vi "Write Start URL.vi"(8 "error in (no error)":errorcluster, 10 "Start URL":string, 11 "WebView2 Control in":refnum<class "WebView2 Control.lvclass">) -> (0 "error out":errorcluster, 3 "WebView2 Control out":refnum<class "WebView2 Control.lvclass">)   [LabVIEW 2020, in "WebView2.lvlib" / "WebView2 Control.lvclass"]
uses:
  WebView2 Control.lvclass
  WebView2 Control.lvclass/WebView2 Control.ctl
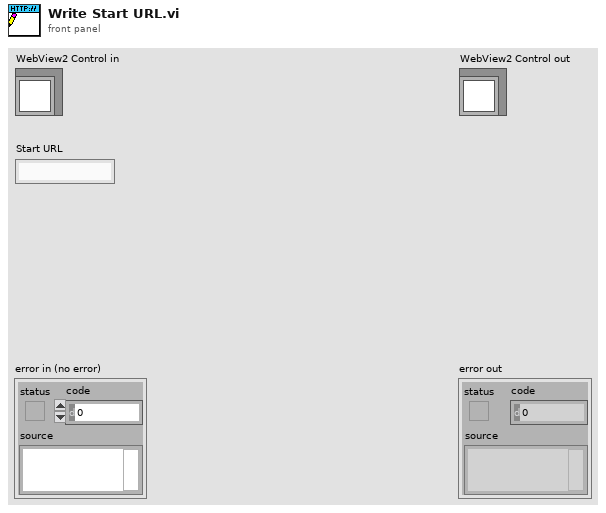
[diagram p1: front panel]
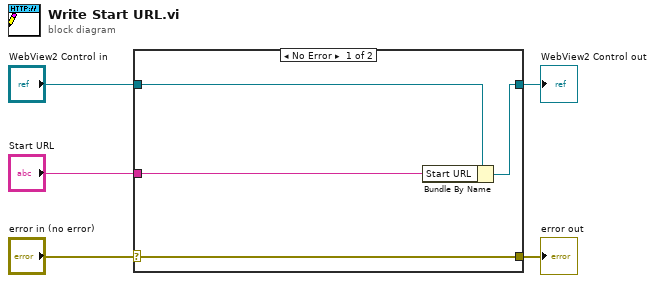
[diagram p0: block diagram]
diagram:
  n1 = case shown="No Error" "error in (no error)" {
    selector: "error in (no error)" -> [w9 w10]
    tunnel: [w9 w10] -> w4
    tunnel: [w7 w11] -> w2
    tunnel: "WebView2 Control in" -> [w8 w11]
    tunnel: "Start URL" -> [w6 _]
    frame No Error {
      n2 = Bundle By Name(cluster=w8, "Start URL"=w6) -> (w7:refnum<class "WebView2 Control.lvclass">)
    }
    frame Error {
    }
  }
  "error out" <- w4
  "WebView2 Control out" <- w2
